vi "Untitled 1.vi"   [LabVIEW 2015]
uses:
  <instrlib>/FlexRIO/Libraries/Adapter Modules/NI 573x/NI 573x CLIP.lvlib
  <instrlib>/FlexRIO/Libraries/Acquisition Engine/Acquisition Engine.lvlib
  <instrlib>/FlexRIO/Libraries/Acquisition Engine/FPGA/Interface/acqEngineTrigger.vi
  <instrlib>/FlexRIO/Libraries/Acquisition Engine/FPGA/Implementation/acqEngineSimpleHistoryFifo-I8.vi
  <instrlib>/FlexRIO/Libraries/Flexible Record Storage/Flexible Record Storage.lvlib
  <instrlib>/FlexRIO/Libraries/Flexible Record Storage/Implementation/Acquisition Storage Mechanism - (BRAM 64-Bit).vi
  <instrlib>/FlexRIO/Libraries/Adapter Modules/NI 5781/NI 5781 CLIP.lvlib
  <instrlib>/FlexRIO/Libraries/Adapter Modules/NI 5761/NI 5761 CLIP.lvlib
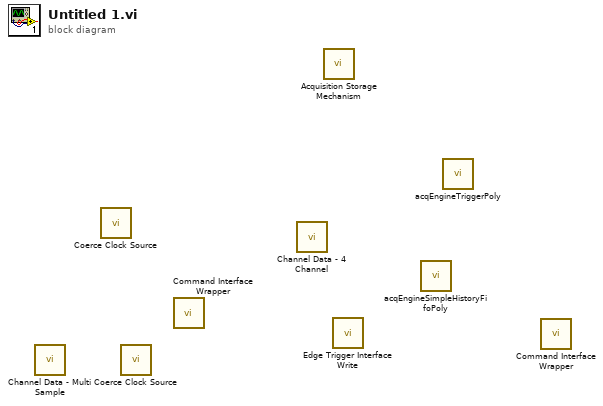
[diagram p0: block diagram]
diagram:
  n1 = call <instrlib>:"Channel Data - Multi Sample.vi"() -> ()  [unwired: 9 in, 3 out]
  n2 = call <instrlib>:"Coerce Clock Source.vi"() -> ()  [unwired: 11 in, 1 out]
  n3 = call <instrlib>:"Coerce Clock Source.vi"() -> ()  [unwired: 11 in, 1 out]
  n4 = call <instrlib>:"Command Interface Wrapper.vi"() -> ()  [unwired: 9 in, 3 out]
  n5 = call <instrlib>:"Channel Data - 4 Channel.vi"() -> ()  [unwired: 9 in, 3 out]
  n6 = call-poly <instrlib>:"Acquisition Storage Mechanism.vi"() -> ()  [unwired: 11 in, 5 out]
  n7 = call <instrlib>:"Edge Trigger Interface Write.vi"() -> ()  [unwired: 12 in]
  n8 = call-poly <instrlib>:"acqEngineSimpleHistoryFifoPoly.vi"() -> ()  [unwired: 9 in, 3 out]
  n9 = call-poly <instrlib>:"acqEngineTriggerPoly.vi"() -> ()  [unwired: 9 in, 3 out]
  n10 = call <instrlib>:"Command Interface Wrapper.vi"() -> ()  [unwired: 9 in, 3 out]
